vi "FTW-Router-Worker.vi"(0 "Backend Handler":refnum<user-event>, 2 "RouterID":i64 format="%016x") -> ()   [LabVIEW 2012, in "FTW-Actor.lvlib" / "FTW-Router.lvclass"]
uses:
  FTW-Router.lvclass
  Request/FTW-Request.lvclass
  Endpoint/FTW-Endpoint.lvclass
panel:
  out "Incoming Message Available":bool
  out "poll err":errorcluster
  out "Message Received?":bool
  out "recv err":errorcluster
  out "Iteration":i32
  out "Incoming Messages":i32
  # "Inputs"
  # "Debug"
  # "Outputs"
  # "This asynchronous worker has no outputs"
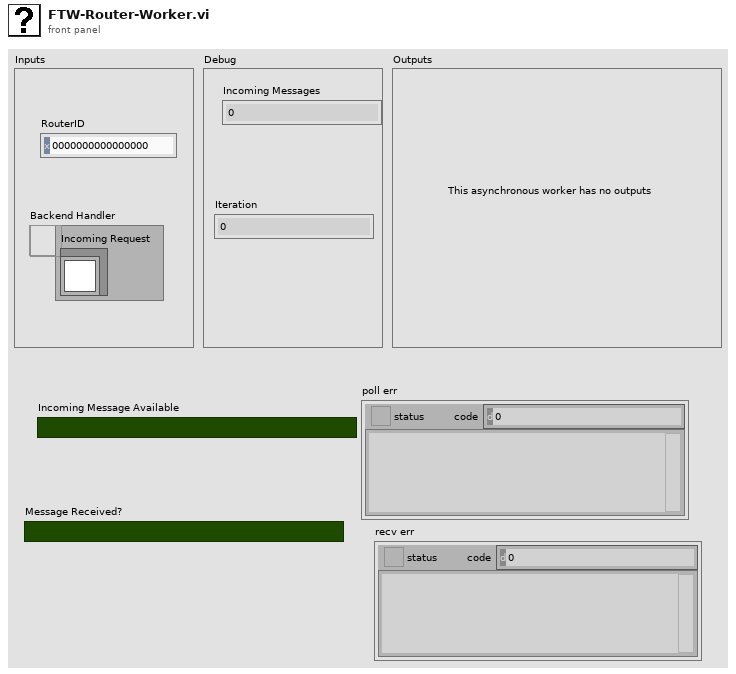
[diagram p1: front panel]
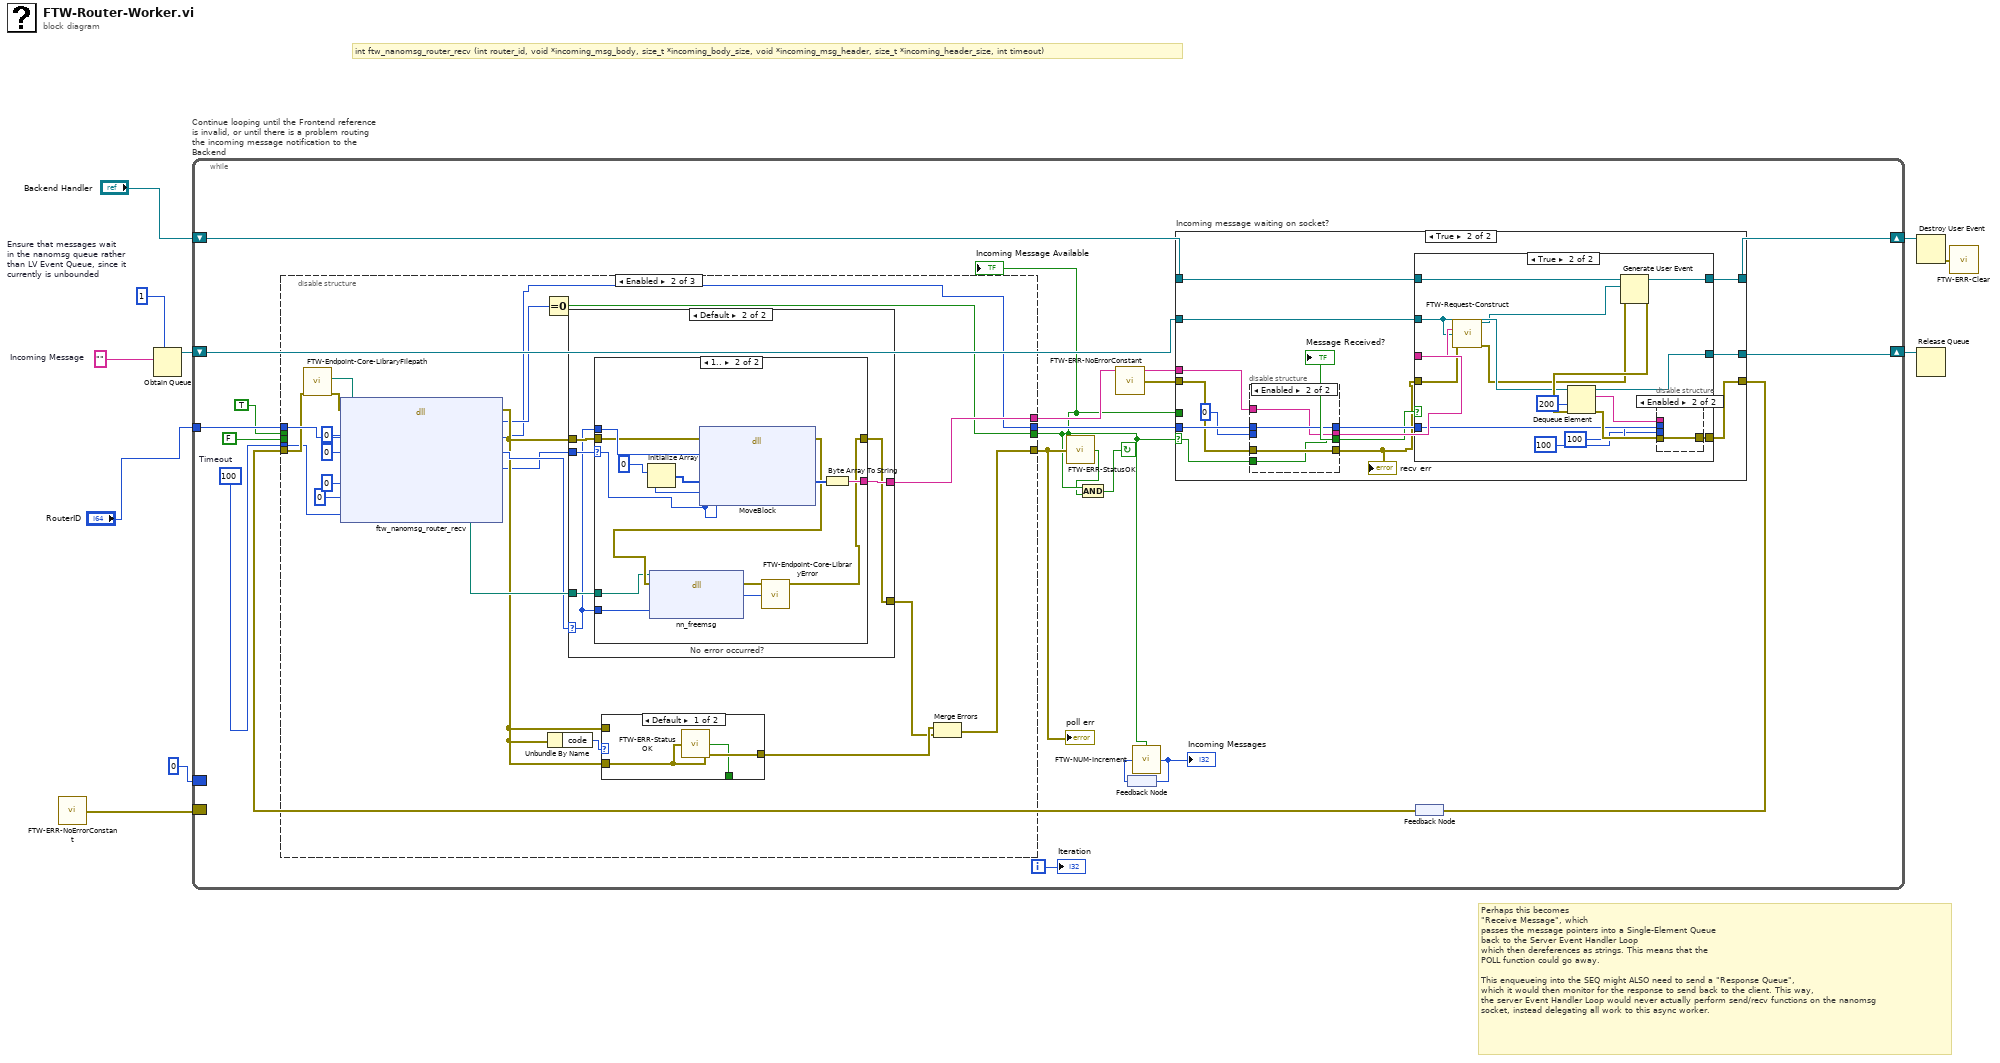
[diagram p0: block diagram]
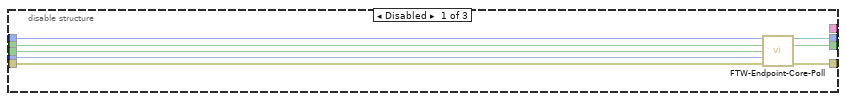
[diagram p2: hidden frame]
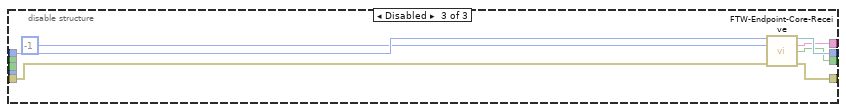
[diagram p6: hidden frame]
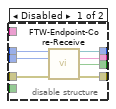
[diagram p8: hidden frame]
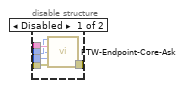
[diagram p10: hidden frame]
diagram:
  w5 = ""  # Incoming Message
  w6 = 1  # Ensure that messages wait in the nanomsg queue rather than LV Event Queue, since it currently is unbounded
  # "int ftw_nanomsg_router_recv (int router_id, void *incoming_msg_body, size_t *incoming_body_size, void *incoming_msg_header, size_t *incoming_header_size, int timeout)"
  # "Perhaps this becomes\n\"Receive Message\", which\npasses the message pointers into a Single-Element Queue\nback to the Server Event Handler Loop\nwhich then dereferences as strings. This means that the\nPOLL function could go away.\n\nThis enqueueing into the SEQ might ALSO need to send a \"Response Queue\",\nwhich it would then monitor for the response to send back to the client. This way,\nthe server Event Handler Loop would never actually perform send/recv functions on the nanomsg\nsocket, instead delegating all work to this async worker."
  n1 = call "FTW-ERR-NoErrorConstant.vi"() -> ("no error"=w2:errorcluster)
  n2 = Obtain Queue(max queue size (-1, unlimited)=w6, element data type=w5) -> (queue out=w7:refnum<queue>)  [unwired: 3 in, 2 out]
  n3 = while "Continue looping until the Frontend reference is invalid, or until there is a problem routing the incoming message notification to the Backend" {
    border: w2 -> [_]
    shift-right: [w28] -> w9
    shift-left: "Backend Handler" -> [w30]
    border: 0 ("Messages Handled") -> [_]
    tunnel: "RouterID" -> [w22]
    shift-right: [w17] -> w3
    shift-left: w7 -> [w25]
    i -> [w26]
    stop <- w11 continue-if-true
    w21 = 100  # Timeout
    n4 = call "FTW-ERR-NoErrorConstant.vi"() -> ("no error"=w27:errorcluster)
    n5 = feedback #1() -> (w23:i32)
    n6 = feedback #2() -> (w19:errorcluster)
    n7 = disable-structure shown="Enabled" {
      disable-tunnel: w22 -> [w39 w55 w91]
      disable-tunnel: w21 -> [w38 w42 _]
      disable-tunnel: [w37 w48 w87] -> w20
      disable-tunnel: w19 -> [w36 w52 w88]
      disable-tunnel: [w35 w43 w90] -> w18
      disable-tunnel: TRUE ("Check for Incoming Messages?") -> [w34 _ _]
      disable-tunnel: FALSE ("Check for Outgoing Messages?") -> [w33 _ _]
      disable-tunnel: [w32 w44 w86] -> w13
      disable-tunnel: [_ w50 w85] -> w14
      frame Disabled {
        n8 = call "FTW-Endpoint-Core-Poll.vi"("FTW Endpoint"=w39, "Check for Incoming Messages?"=w34, "Check for Outgoing Messages?"=w33, "Timeout"=w38, "error in"=w36) -> ("FTW Endpoint out"=w35:refnum<class "FTW-Endpoint.lvclass">, "Incoming Message Available"=w32:bool, "Outgoing Message Available"=w31:bool, "error out"=w37:errorcluster)  [unwired: 7 in]
      }
      frame Enabled {
        n9 = call "FTW-Endpoint-Core-LibraryFilepath.vi"("error in"=w52) -> ("error out"=w54:errorcluster, "Library Filepath"=w53:path)  [unwired: 8 in, 1 out]
        n10 = dll-call lib="?" fn="ftw_nanomsg_router_recv"(path in=w53, error in=w54, "RouterID"=w55, "Message Body Pointer"=i64 0, "Message Body Length"=u64 0, "Message Header Pointer"=i64 0, "Message Header Length"=u64 0, "Timeout"=w42) -> (path out=w57:path, error out=w51:errorcluster, "Return Value"=w45:i64, "RouterID"=w43:i64, "Message Body Pointer"=w56:i64, "Message Body Length"=w49:u64)  [unwired: 4 in]
        n11 = Equal To 0?(x=w45) -> (x = 0?=w44:bool)
        n12 = Unbundle By Name(w51) -> ("code"=w60:i32)
        n13 = case shown="Default" w56 {
          selector: w56 -> [_ w62]
          tunnel: [w61 w64] -> w58
          tunnel: w57 -> [_ w63]
          tunnel: w49 -> [_ w67]
          tunnel: [_ w66] -> w50
          tunnel: w51 -> [w61 w65]
          frame 0 {
          }
          frame Default {
            n14 = case "No error occurred?" shown="1.." w67 {
              selector: w67 -> [_ w75]
              tunnel: [w68 w69] -> w64
              tunnel: [_ w76] -> w66
              tunnel: w62 -> [_ w81]
              tunnel: w65 -> [w68 w79]
              tunnel: w63 -> [_ w73]
              tunnel: w62 -> [_ w72]
              frame ..0 {
              }
              frame 1.. {
                n15 = Initialize Array(u8 0, w75) -> (w78:u8[])
                n16 = dll-call lib="LabVIEW" fn="MoveBlock"(error in=w79, "Source Pointer"=w81, "Pointer to Destination"=w78, "String Length"=w75) -> (error out=w74:errorcluster, "Pointer to Destination"=w77:u8[])  [unwired: 5 in, 1 out]
                n17 = dll-call lib="?" fn="nn_freemsg"(path in=w73, error in=w74, "Message Pointer"=w72) -> (error out=w71:errorcluster, "Return Value"=w70:i64)  [unwired: 2 in, 1 out]
                n18 = call "FTW-Endpoint-Core-LibraryError.vi"("error in"=w71, "Return Value"=w70) -> ("error out"=w69:errorcluster)  [unwired: 13 in]
                n19 = Byte Array To String(unsigned byte array=w77) -> (string=w76:string)
              }
            }
          }
        }
        n20 = case shown="Default" w60 {
          tunnel: [w83 w84] -> w59
          tunnel: w51 -> [w83 _]
          tunnel: w51 -> [_ w84]
          tunnel: [w82 _] -> _
          frame Default {
            n21 = call "FTW-ERR-StatusOK.vi"("error to check"=w83) -> ("Status OK?"=w82:bool)
          }
          frame 11 {
          }
        }
        n22 = Merge Errors(w59, w58) -> (w48:errorcluster)
      }
      frame Disabled {
        n23 = call "FTW-Endpoint-Core-Receive.vi"("FTW Endpoint"=w91, "Timeout"=-1, "error in"=w88) -> ("FTW Endpoint out"=w90:refnum<class "FTW-Endpoint.lvclass">, "Message"=w85:string, "Message Received?"=w86:bool, "error out"=w87:errorcluster)  [unwired: 7 in, 2 out]
      }
    }
    "poll err" <- w20
    "Incoming Message Available" <- w13
    n24 = call "FTW-ERR-StatusOK.vi"("error to check"=w20) -> ("Status OK?"=w12:bool)
    n25 = And(x=w13, y=w12) -> (x .and. y?=w11:bool)
    n26 = call "FTW-NUM-Increment.vi"("Initial Value"=w23, "Increment?"=w13) -> ("Final Value"=w24:i32)
    "Incoming Messages" <- w24
    n27 = feedback-in #1(w24) -> ()
    n28 = case "Incoming message waiting on socket?" shown="True" w13 {
      selector: w13 -> [_ w95]
      tunnel: w30 -> [w94 w108]
      tunnel: [w93 w105] -> w29
      tunnel: [w94 w107] -> w28
      tunnel: w27 -> [w93 w102]
      tunnel: w18 -> [_ w103]
      tunnel: w25 -> [w92 w106]
      tunnel: w13 -> [_ _]
      tunnel: [w92 w104] -> w17
      tunnel: w14 -> [_ w96]
      frame False {
      }
      frame True {
        n29 = disable-structure shown="Enabled" {
          disable-tunnel: w103 -> [w115 w119]
          disable-tunnel: w102 -> [w114 w118]
          disable-tunnel: 0 ("Timeout") -> [w113 _]
          disable-tunnel: [w112 w119] -> w100
          disable-tunnel: [w111 w117] -> w99
          disable-tunnel: [w110 w116] -> w98
          disable-tunnel: [w109 w118] -> w97
          disable-tunnel: w96 -> [_ w117]
          disable-tunnel: w95 -> [_ w116]
          frame Disabled {
            n30 = call "FTW-Endpoint-Core-Receive.vi"("FTW Endpoint"=w115, "Timeout"=w113, "error in"=w114) -> ("FTW Endpoint out"=w112:refnum<class "FTW-Endpoint.lvclass">, "Message"=w111:string, "Message Received?"=w110:bool, "error out"=w109:errorcluster)  [unwired: 7 in, 2 out]
          }
          frame Enabled {
          }
        }
        "recv err" <- w97
        "Message Received?" <- w98
        n31 = case shown="True" w98 {
          tunnel: w108 -> [w122 w138]
          tunnel: [w122 w137] -> w107
          tunnel: w106 -> [w121 w128]
          tunnel: [w120 w134] -> w105
          tunnel: [w121 w131] -> w104
          tunnel: w97 -> [w120 w126]
          tunnel: w100 -> [_ w130]
          tunnel: w99 -> [_ w129]
          frame False {
          }
          frame True {
            n32 = call "FTW-Request-Construct.vi"("Verbatim Request"=w129, "Response Broker"=w128, "error in"=w126) -> ("FTW Request out"=w127:refnum<class "FTW-Request.lvclass">, "error out"=w125:errorcluster)  [unwired: 11 in]
            n33 = Generate User Event(user event=w138, event data cluster=w127, error in=w125) -> (user event out=w137:refnum<user-event>, error out=w135:errorcluster)
            n34 = Dequeue Element(queue=w128, timeout in ms (-1)=200, error in (no error)=w135) -> (queue out=w131:refnum<queue>, element=w133:string, error out=w136:errorcluster)  [unwired: 1 out]
            n35 = disable-structure shown="Enabled" {
              disable-tunnel: w136 -> [w144 w145]
              disable-tunnel: [w143 w145] -> w134
              disable-tunnel: w133 -> [w142 _]
              disable-tunnel: w130 -> [w141 _]
              disable-tunnel: 100 ("Read Timeout") -> [w140 _]
              disable-tunnel: 100 ("Write Timeout") -> [w139 _]
              frame Disabled {
                n36 = call "FTW-Endpoint-Core-Ask.vi"("FTW Socket"=w141, "Request"=w142, "Read Timeout"=w140, "Write Timeout"=w139, "error in"=w144) -> ("error out"=w143:errorcluster)  [unwired: 6 in, 4 out]
              }
              frame Enabled {
              }
            }
          }
        }
      }
    }
    n37 = feedback-in #2(w29) -> ()
    "Iteration" <- w26
  }
  n38 = Destroy User Event(user event=w9) -> (error out=w4:errorcluster)  [unwired: 1 in]
  n39 = Release Queue(queue=w3) -> ()  [unwired: 2 in, 3 out]
  n40 = call "FTW-ERR-Clear.vi"("error to snuff"=w4) -> ()  [unwired: 1 out]
